vi "SiosIfmSetPreset.vi"(1 "Value":dbl, 2 "Channel":i32, 3 "Device Number":i32) -> (0 "Success":i32)   [LabVIEW 2009]
uses:
  siosifm.dll
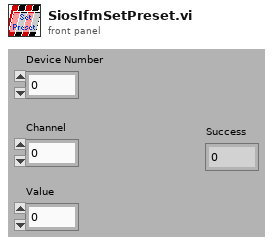
[diagram p1: front panel]
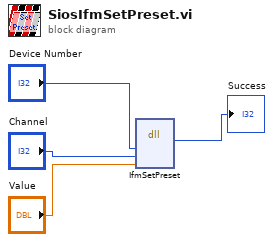
[diagram p0: block diagram]
diagram:
  n1 = dll-call lib="C:/WORK/Artem/RE-10/SIOS_IfmDLL/siosifm.dll" fn="IfmSetPreset"("devNumber"="Device Number", "channel"="Channel", "presetValue"="Value") -> ("success"=→"Success":i32)  [unwired: 6 in, 2 out]
